vi "gfitsio-write-image-subset-variant.vi"(6 "fpixel":i32[](array[numeric]), 8 "error in (no error)":errorcluster, 9 "data":variant, 11 "gfits refnum":T1) -> (0 "error out":errorcluster, 3 "dup gfits refnum":T1)   [LabVIEW 2014, in "gfitsio.lvlib"]
doc: "Write to a subset of the FITS data array. <B>fpixel</B> specifies the first pixel in the subset and must have the same number of elements as the image has dimensions. The data array will be written along the fastest changing dimensions of the image. This starts with NAXIS1 in the FITS file (column-major order) and in LabVIEW this starts with the last element in <b>fpixel</b> (row-major order)."
uses:
  gfitsio/gfitsio.lvlib
  gfitsio-refnum.ctl
  gfitsio/gfitsio.dll
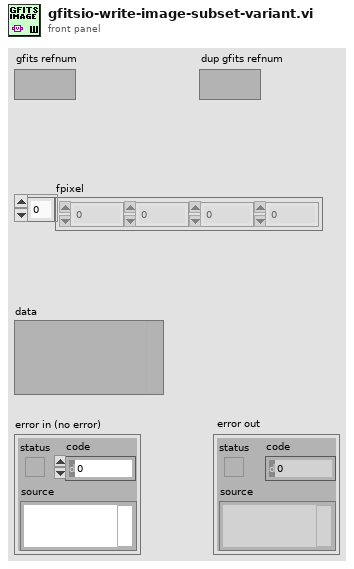
[diagram p1: front panel]
types:
  T1 = typedef "gfitsio.lvlib/gfitsio-refnum.ctl" = refnum<k1>
  T2 = typedef "gfitsio.lvlib/cfitsio-datatypes.ctl" = i32
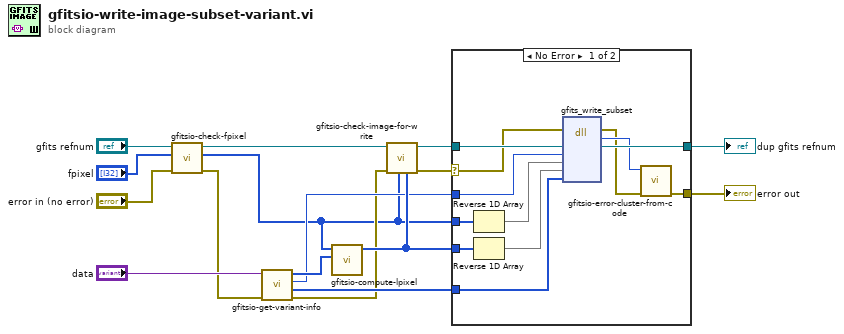
[diagram p0: block diagram]
diagram:
  n1 = call "gfitsio-check-fpixel.vi"("error in (no error)"="error in (no error)", "fpixel"="fpixel", "gfits refnum"="gfits refnum") -> ("error out"=w3:errorcluster, "fpixel out"=w1:i32[], "dup gfits refnum"=w5:T1)  [unwired: 6 in]
  n2 = call "gfitsio-get-variant-info.vi"("error in (no error)"=w3, "variant"="data") -> ("error out"=w8:errorcluster, "data out"=w9:u8[], "cfitsio datatype"=w10:T2, "sizes"=w12:i32[])  [unwired: 6 in]
  n3 = call "gfitsio-compute-lpixel.vi"("dimension sizes of subset"=w12, "fpixel in"=w1) -> ("lpixel"=w11:i32[])  [unwired: 9 in]
  n4 = call "gfitsio-check-image-for-write.vi"("lpixel"=w11, "fpixel"=w1, "error in (no error)"=w8, "gfits refnum"=w5) -> ("error out"=w7:errorcluster, "dup gfits refnum"=w14:T1)  [unwired: 6 in]
  n5 = case shown="No Error" w7 {
    selector: w7 -> [w17 w30]
    tunnel: [w28 w30] -> w16
    tunnel: [w26 w29] -> w15
    tunnel: w14 -> [w27 w29]
    tunnel: w1 -> [w21 _]
    tunnel: w11 -> [w24 _]
    tunnel: w10 -> [w20 _]
    tunnel: w9 -> [w19 _]
    frame No Error {
      n6 = Reverse 1D Array(array=w21) -> (reversed array=w22:i32[])
      n7 = Reverse 1D Array(array=w24) -> (reversed array=w23:i32[])
      n8 = dll-call lib="F:/labview_codes/labview_codes/gfitsio/gfitsio.dll" fn="gfits_write_subset"(error in=w17, "refnum"=w27, "datatype"=w20, "fpixel"=w22, "lpixel"=w23, "array"=w19) -> (error out=w18:errorcluster, "return type"=w25:i32, "refnum"=w26:T1)  [unwired: 4 in, 3 out]
      n9 = call "gfitsio-error-cluster-from-code.vi"("error in (no error)"=w18, "error code"=w25) -> ("error out"=w28:errorcluster)  [unwired: 9 out]
    }
    frame Error {
    }
  }
  "error out" <- w16
  "dup gfits refnum" <- w15
